vi "NewCore.vi"(8 "error in (no error)":errorcluster, 10 "ParamsArray":variant[](array[variant]), 11 "Door":refnum<class "Door.lvclass">) -> (0 "error out":errorcluster, 3 "Door":refnum<class "Door.lvclass">)   [LabVIEW 2020, in "Door.lvclass"]
uses:
  Door.lvclass
  TypeDef/DoorParams.ctl
  Room/Room.lvclass
  Private/TypeDef/privateData.ctl
  Door.lvclass/Door.ctl
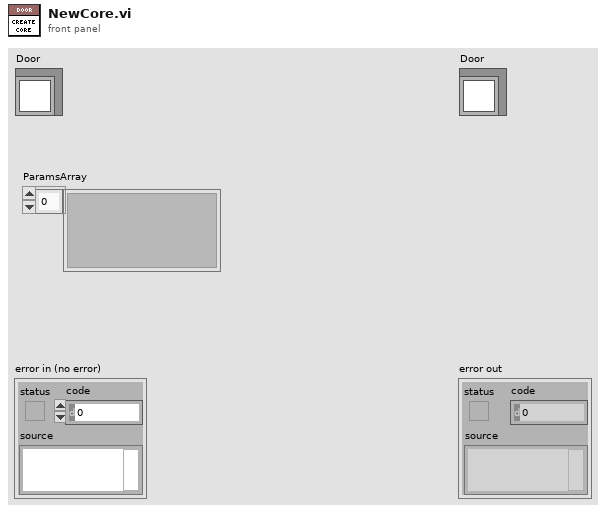
[diagram p1: front panel]
types:
  T1 = typedef "Door.lvclass/privateData.ctl" = cluster{"room1":refnum<class "Room.lvclass">, "room2":refnum<class "Room.lvclass">}
  T2 = typedef "Door.lvclass/DoorParams.ctl" = cluster{"room1":refnum<class "Room.lvclass">, "room2":refnum<class "Room.lvclass">}
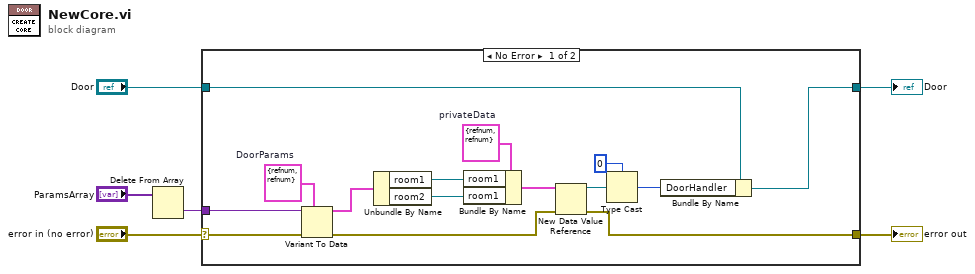
[diagram p0: block diagram]
diagram:
  n1 = Delete From Array(array="ParamsArray") -> (deleted portion=w3:variant)  [unwired: 2 in, 1 out]
  n2 = case shown="No Error" "error in (no error)" {
    selector: "error in (no error)" -> [w14 w23]
    tunnel: [w16 w23] -> w5
    tunnel: [w18 w22] -> w6
    tunnel: "Door" -> [w17 w22]
    tunnel: w3 -> [w12 _]
    frame No Error {
      w10 = T1 {"room1"=refnum, "room2"=refnum}  # privateData
      w15 = T2 {"room1"=refnum, "room2"=refnum}  # DoorParams
      n3 = Variant To Data(error in=w14, type=w15, Variant=w12) -> (data=w11:T2, error out=w13:errorcluster)
      n4 = Unbundle By Name(w11) -> ("room1"=w8:refnum<class "Room.lvclass">, "room2"=w9:refnum<class "Room.lvclass">)
      n5 = Bundle By Name(cluster=w10, "room1"=w8, "room1"=w9) -> (w7:T1)
      n6 = New Data Value Reference(data value=w7, error in=w13) -> (data value reference=w21:refnum<data-value>, error out=w16:errorcluster)
      n7 = Type Cast(type=u32 0, x=w21) -> (*(type *) &x=w19:u32)
      n8 = Bundle By Name(cluster=w17, "DoorHandler"=w19) -> (w18:refnum<class "Door.lvclass">)
    }
    frame Error {
    }
  }
  "error out" <- w5
  "Door" <- w6
